vi "Read EventData.vi"(8 "error in (no error)":errorcluster, 11 "Event in":refnum<class "Event.lvclass">) -> (0 "error out":errorcluster, 2 "EventData":cluster{"Classification":T1}, 3 "Event out":refnum<class "Event.lvclass">)   [LabVIEW 2019, in "Event.lvclass"]
uses:
  Event.lvclass
  TypeDef/Event Classification.ctl
  Event.lvclass/Event.ctl
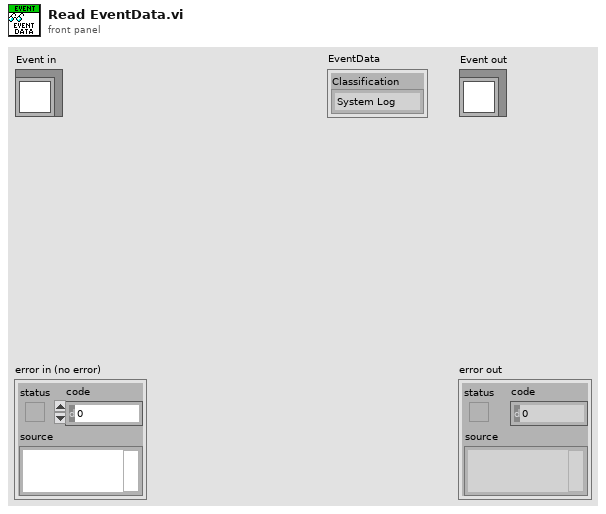
[diagram p1: front panel]
types:
  T1 = typedef "Event.lvclass/Event Classification.ctl" = enum16{"System Log", "test1", "test2", "test3"}
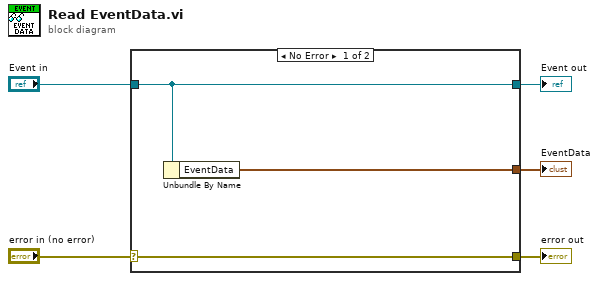
[diagram p0: block diagram]
diagram:
  n1 = case shown="No Error" "error in (no error)" {
    selector: "error in (no error)" -> [w8 w9]
    tunnel: [w8 w9] -> w4
    tunnel: [w7 w10] -> w2
    tunnel: "Event in" -> [w7 w10]
    tunnel: [w6 _] -> w1
    frame No Error {
      n2 = Unbundle By Name(w7) -> ("EventData"=w6:cluster{"Classification":T1})
    }
    frame Error {
    }
  }
  "error out" <- w4
  "Event out" <- w2
  "EventData" <- w1
